vi "zadanie3.vi"() -> ()   [LabVIEW 2023]
panel:
  out "Array":bool[][](array[boolean])
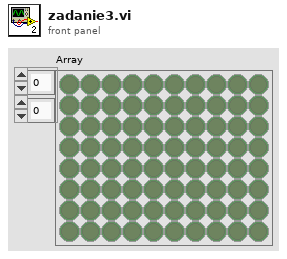
[diagram p1: front panel]
types:
  T1 = enum16{"open", "replace", "create", "open or create", "replace or create", "replace or create with confirmation"}
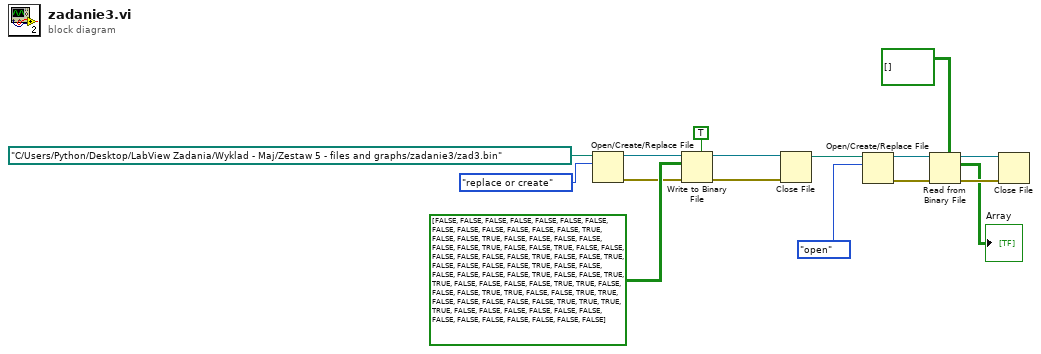
[diagram p0: block diagram]
diagram:
  n1 = Open/Create/Replace File(file path (use dialog)=path "C:/Users/Python/Desktop/LabView Zadania/Wyklad - Maj/Zestaw 5 - files and graphs/zadanie3/zad3.bin", operation (0:open)=T1."replace or create") -> (refnum out=w15:refnum<file>, error out=w11:errorcluster)  [unwired: 4 in, 1 out]
  n2 = Write to Binary File(file (use dialog)=w15, data=bool[][] [[FALSE, FALSE, FALSE, FALSE, FALSE, FALSE, FALSE, FALSE, FALSE, FALSE], [FALSE, FALSE, FALSE, TRUE, FALSE, FALSE, TRUE, FALSE, FALSE, FALSE], [FALSE, FALSE, FALSE, TRUE, FALSE, FALSE, TRUE, FALSE, FALSE, FALSE], [FALSE, FALSE, FALSE, TRUE, FALSE, FALSE, TRUE, FALSE, FALSE, FALSE], [FALSE, TRUE, FALSE, FALSE, FALSE, FALSE, FALSE, FALSE, TRUE, FALSE], [FALSE, TRUE, TRUE, FALSE, FALSE, FALSE, FALSE, TRUE, TRUE, FALSE], [FALSE, FALSE, TRUE, TRUE, FALSE, FALSE, TRUE, TRUE, FALSE, FALSE], [FALSE, FALSE, FALSE, TRUE, TRUE, TRUE, TRUE, FALSE, FALSE, FALSE], [FALSE, FALSE, FALSE, FALSE, FALSE, FALSE, FALSE, FALSE, FALSE, FALSE]] ("Array"), error in=w11, 5:TRUE ("prepend array or string size? (T)")) -> (refnum out=w14:refnum<file>, error out=w10:errorcluster)  [unwired: 2 in, 1 out]
  n3 = Close File(refnum=w14, error in=w10) -> (path=w3:path)  [unwired: 1 out]
  n4 = Open/Create/Replace File(file path (use dialog)=w3, operation (0:open)=T1."open") -> (refnum out=w9:refnum<file>, error out=w8:errorcluster)  [unwired: 4 in, 1 out]
  n5 = Read from Binary File(5:bool[][] [] ("Boolean"), 8:w8, 11:w9) -> (0:w6:errorcluster, 2:→"Array":bool[][], 3:w7:refnum<file>)  [unwired: 3 in, 1 out]
  n6 = Close File(refnum=w7, error in=w6) -> ()  [unwired: 2 out]
